vi "obj_LuaVIEW Task List_srv.vi"(0 "method":T4, 7 "certificate":string, 11 "task identifier":string) -> (6 "task info list":T1[](array[typedef]) {"handle mask" format="%.0b"; "allow mask" format="%.0b"; "signal flags" format="%.0b"}, 15 "error out":errorcluster)   [LabVIEW 2012]
doc: "A wrapper around the task list object that provides secured remote access to a subset of its methods."
uses:
  typedefs/t_LuaVIEW Served Task List Methods.ctl
  typedefs/clusters/LuaVIEW Task Info.ctl
  typedefs/t_LuaVIEW Task Modes.ctl
  typedefs/t_LuaVIEW Reference.ctl
  clientsrv/typedefs/t_ClientSrv Access Levels.ctl
  typedefs/t_LuaVIEW Task List Methods.ctl
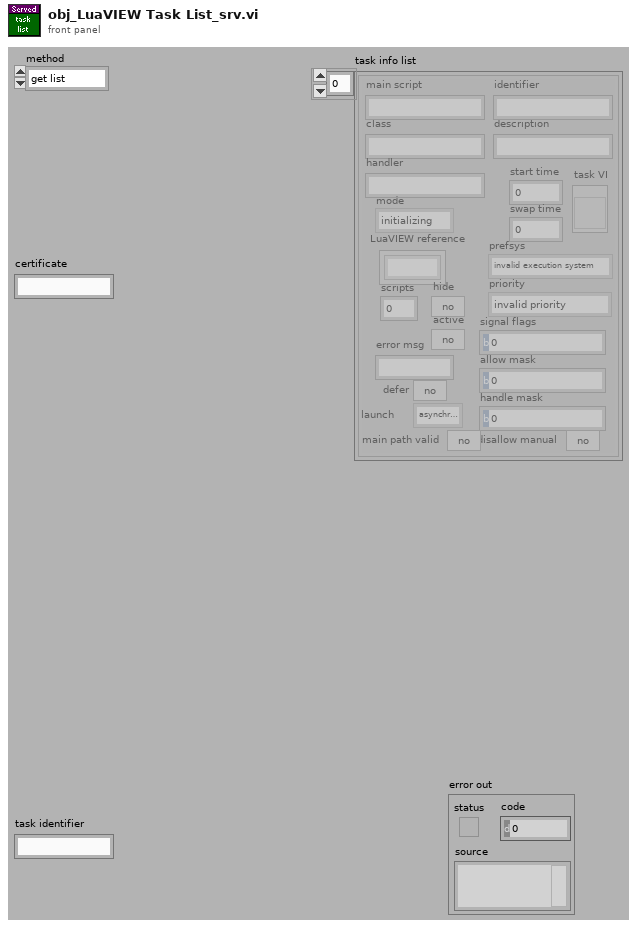
[diagram p1: front panel]
types:
  T1 = typedef "LuaVIEW Task Info.ctl" = cluster{"main script":string, "identifier":string, "class":string, "description":string, "mode":T2, "handler":string, "LuaVIEW reference":T3, "scripts":i32, "hide":bool, "active":bool, "error msg":string, "defer":bool, "launch":enum16{"asynchronous", "manual", "synchronous"}, "main path valid":bool, "start time":dbl, "swap time":dbl, "task VI":refnum<vi>, "prefsys":enum32{"invalid execution system", "user interface", "standard", "instrument i/o", "data acquisition", "other 1", "other 2", "same as caller"}, "priority":enum32{"invalid priority", "background priority", "normal priority", "above normal priority", "high priority", "time critical priority", "subroutine"}, "signal flags":u32, "allow mask":u32, "handle mask":u32, "disallow manual":bool}
  T2 = typedef "t_LuaVIEW Task Modes.ctl" = enum16{"initializing", "running", "executing", "paused", "error", "swapping"}
  T3 = typedef "t_LuaVIEW Reference.ctl" = refnum<k1>
  T4 = typedef "t_LuaVIEW Served Task List Methods.ctl" = enum16{"get list", "resume", "pause", "swap", "stop", "confirm"}
  T5 = typedef "t_ClientSrv Access Levels.ctl" = enum16{"observer", "operator", "local"}
  T6 = typedef "t_LuaVIEW Task List Methods.ctl" = enum16{"clear list", "add", "test", "remove", "get ref", "get task info", "get list", "get script info", "ongoing?", "resume", "pause", "stop", "confirm", "message"}
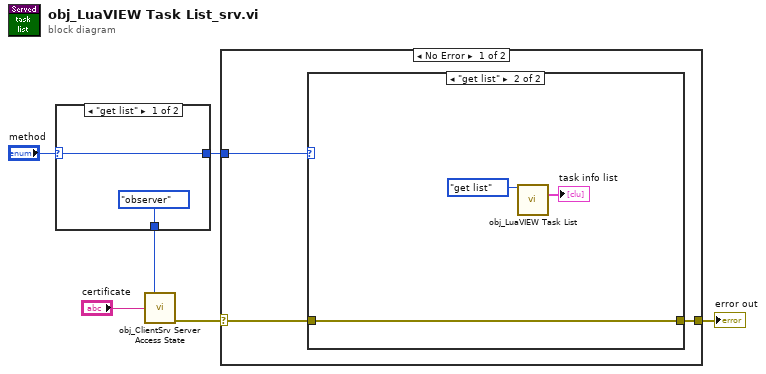
[diagram p0: block diagram]
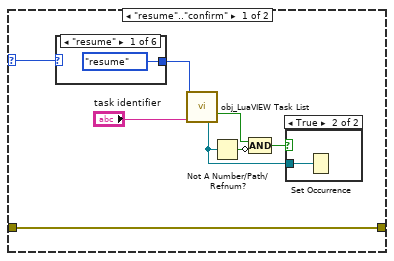
[diagram p2: hidden frame]
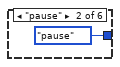
[diagram p3: hidden frame]
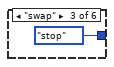
[diagram p4: hidden frame]
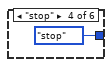
[diagram p5: hidden frame]
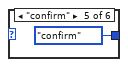
[diagram p6: hidden frame]
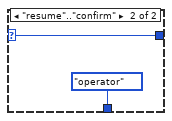
[diagram p10: hidden frame]
diagram:
  n1 = case shown="\"get list\"" "method" {
    selector: "method" -> [w7 w10]
    tunnel: [w7 w10] -> w4
    tunnel: [t_ClientSrv_Access_Levels."observer" ("access level") t_ClientSrv_Access_Levels."operator" ("access level")] -> w2
    frame "get list" {
    }
    frame "resume".."confirm" {
    }
  }
  n2 = call "obj_ClientSrv Server Access State.vi"("access level"=w2, "certificate in"="certificate") -> ("error out"=w3:errorcluster)  [unwired: 11 in, 2 out]
  n3 = case shown="No Error" w3 {
    selector: w3 -> [w12 w31]
    tunnel: [w11 w31] -> w5
    tunnel: w4 -> [w13 _]
    frame No Error {
      n4 = case shown="\"get list\"" w13 {
        selector: w13 -> [w16 _]
        tunnel: w12 -> [w15 w28]
        tunnel: [w15 w28] -> w11
        frame "resume".."confirm" {
          n5 = case shown="\"resume\"" w16 {
            tunnel: [t_LuaVIEW_Task_List_Methods."resume" ("method") t_LuaVIEW_Task_List_Methods."pause" ("method") t_LuaVIEW_Task_List_Methods."stop" ("method") t_LuaVIEW_Task_List_Methods."stop" ("method") t_LuaVIEW_Task_List_Methods."confirm" ("method") _] -> w17
            frame "resume" {
            }
            frame "pause" {
            }
            frame "swap" {
            }
            frame "stop" {
            }
            frame "confirm" {
            }
            frame Default {
            }
          }
          n6 = call "obj_LuaVIEW Task List.vi"("method"=w17, "task identifier"="task identifier") -> ("set/ongoing"=w21:bool, "wakeup occurrence"=w18:refnum<k4>)  [unwired: 8 in, 4 out]
          n7 = Not A Number/Path/Refnum?(number/path/refnum=w18) -> (NaN/Path/Refnum?=w20:bool)
          n8 = Compound Arithmetic op=AND(w21, invert w20) -> (w19:bool)
          n9 = case shown="True" w19 {
            tunnel: w18 -> [_ w27]
            frame False {
            }
            frame True {
              n10 = Set Occurrence(w27) -> ()
            }
          }
        }
        frame "get list" {
          n11 = call "obj_LuaVIEW Task List.vi"("method"=t_LuaVIEW_Task_List_Methods."get list") -> ("task info list"=→"task info list":T1[])  [unwired: 9 in, 5 out]
        }
      }
    }
    frame Error {
    }
  }
  "error out" <- w5
